vi "solar_voy Get Info (SEQ).vi"(10 "Voyager SEQ in":refnum<queue>) -> (1 "Interface Name":string, 2 "Voyager SEQ out":refnum<queue>, 5 "Valid?":bool)   [LabVIEW 2018]
doc: "This returns the Voyager interface name."
uses:
  solar_voy_def/solar_voy_def_ctl PACKET_ID.ctl
  solar_voy_ctl Voyager.ctl
  solar_voy_def/solar_voy_def_ctl ITEM TYPE.ctl
  type/solar_type Item Type.ctl
  solar_voy_def/solar_voy_def_ctl ITEM.ctl
  solar_voy_def/solar_voy_def_ctl PACKET.ctl
  solar_voy_def/solar_voy_def_ctl HDR.ctl
  solar_voy_ctl TCP.ctl
  solar_voy_ctl Port Setup.ctl
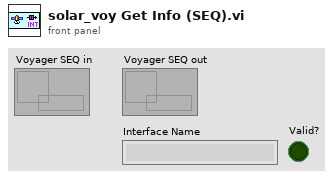
[diagram p1: front panel]
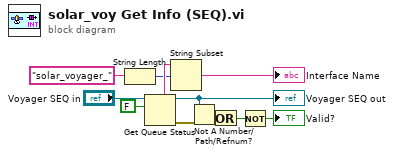
[diagram p0: block diagram]
diagram:
  n1 = String Length(string="solar_voyager_" ("regular expression")) -> (length=w8:i32)
  n2 = Get Queue Status(queue="Voyager SEQ in", return elements? (F)=FALSE) -> (queue out=w1:refnum<queue>, queue name=w10:string, error out=w5:errorcluster)  [unwired: 1 in, 5 out]
  "Voyager SEQ out" <- w1
  n3 = String Subset(string=w10, offset (0)=w8) -> (substring=→"Interface Name":string)  [unwired: 1 in]
  n4 = Not A Number/Path/Refnum?(number/path/refnum=w1) -> (NaN/Path/Refnum?=w6:bool)
  n5 = Or(x=w6, y=w5) -> (x .or. y?=w4:bool)
  n6 = Not(x=w4) -> (.not. x?=→"Valid?":bool)
